vi "LineAlg.vi"(10 "array":bool[](array[boolean]), 11 "Kp":dbl) -> (1 "logical OR":bool, 3 "appended array":dbl[](array[numeric]))   [LabVIEW 2019]
panel:
  in  "y 3":i16=100
  in  "y":i16=470
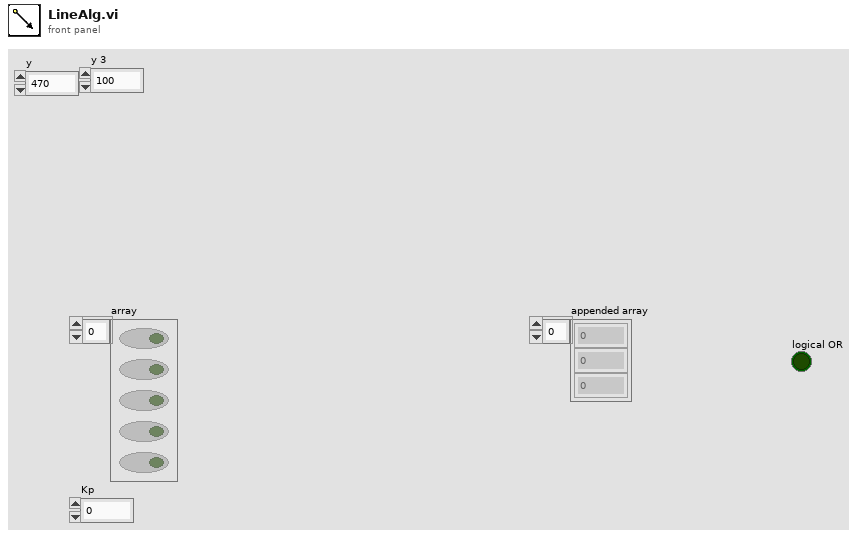
[diagram p1: front panel]
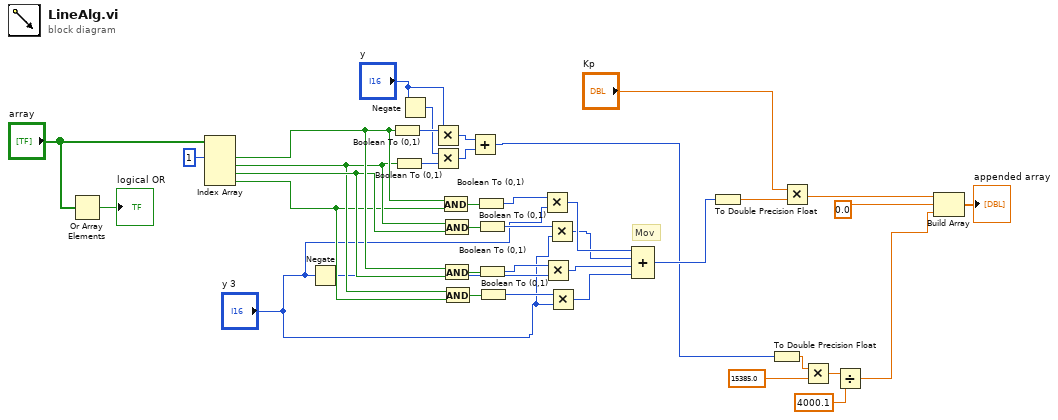
[diagram p0: block diagram]
diagram:
  # "Mov"
  n1 = Or Array Elements(Boolean array="array") -> (logical OR=→"logical OR":bool)
  n2 = Index Array(array="array", index #1=1 ("index")) -> (element #1=w24:bool, element #2=w22:bool, element #3=w23:bool, element #4=w21:bool)  [unwired: 3 in]
  n3 = Negate(x="y 3") -> (-x=w6:i16)
  n4 = Boolean To (0,1)(Boolean=w24) -> (0, 1=w32:i16)
  n5 = Boolean To (0,1)(Boolean=w22) -> (0, 1=w31:i16)
  n6 = Negate(x="y") -> (-x=w9:i16)
  n7 = Multiply(x=w32, y="y") -> (x*y=w29:i16)
  n8 = Multiply(x=w9, y=w31) -> (x*y=w30:i16)
  n9 = And(x=w24, y=w21) -> (x .and. y?=w27:bool)
  n10 = And(x=w22, y=w23) -> (x .and. y?=w28:bool)
  n11 = And(x=w24, y=w23) -> (x .and. y?=w8:bool)
  n12 = And(x=w22, y=w21) -> (x .and. y?=w7:bool)
  n13 = Add(x=w29, y=w30) -> (x+y=w3:i16)
  n14 = Boolean To (0,1)(Boolean=w27) -> (0, 1=w12:i16)
  n15 = Boolean To (0,1)(Boolean=w28) -> (0, 1=w11:i16)
  n16 = Boolean To (0,1)(Boolean=w8) -> (0, 1=w25:i16)
  n17 = Boolean To (0,1)(Boolean=w7) -> (0, 1=w26:i16)
  n18 = Multiply(x=w12, y="y 3") -> (x*y=w14:i16)
  n19 = Multiply(x=w25, y=w6) -> (x*y=w20:i16)
  n20 = Multiply(x=w11, y="y 3") -> (x*y=w13:i16)
  n21 = Multiply(x=w26, y="y 3") -> (x*y=w19:i16)
  n22 = Compound Arithmetic op=ADD(w14, w13, w20, w19) -> (w18:i16)
  n23 = To Double Precision Float(number=w18) -> (double precision float=w17:dbl)
  n24 = To Double Precision Float(number=w3) -> (double precision float=w2:dbl)
  n25 = Multiply(x="Kp", y=w17) -> (x*y=w16:dbl)
  n26 = Multiply(x=w2, y=15385.0) -> (x*y=w34:dbl)
  n27 = Divide(x=w34, y=4000.1) -> (x/y=w1:dbl)
  n28 = Build Array(w16, 0.0 ("element"), w1) -> (→"appended array":dbl[])
